vi "Get Session ID.vi"(11 "WelcomeHandler JSON in":refnum<class "WelcomeHandler JSON.lvclass">) -> (2 "Session ID":u64, 3 "WelcomeHandler JSON out":refnum<class "WelcomeHandler JSON.lvclass">)   [LabVIEW 2020, in "wamplv.lvlib" / "WelcomeHandler JSON.lvclass"]
uses:
  WelcomeHandler JSON.lvclass
  WelcomeHandler JSON.lvclass/WelcomeHandler JSON.ctl
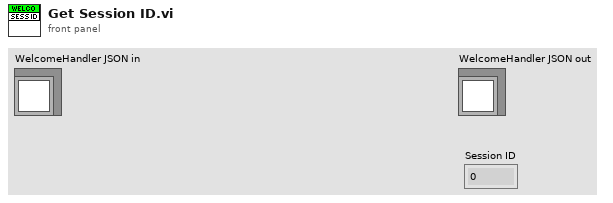
[diagram p1: front panel]
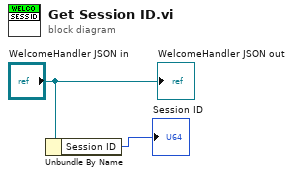
[diagram p0: block diagram]
diagram:
  n1 = Unbundle By Name("WelcomeHandler JSON in") -> ("Session ID"=→"Session ID":u64)
  "WelcomeHandler JSON out" <- "WelcomeHandler JSON in"
